vi "RandomInt64.vi"(10 "Min":i64, 11 "Max":i64) -> (3 "Random":i64)   [LabVIEW 2013]
doc: "Gives a random number between the two inputs, inclusive. \"Max\" can actually be smaller than \"Min,\" in this case, a random number [Max, Min] is given."
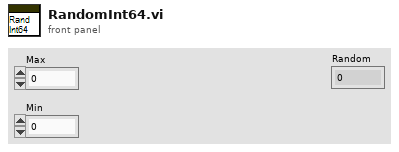
[diagram p1: front panel]
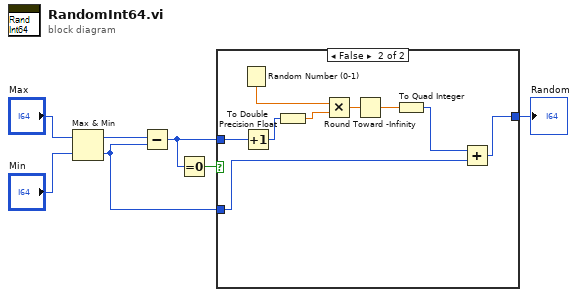
[diagram p0: block diagram]
diagram:
  n1 = Max & Min(x="Max", y="Min") -> (max(x,y)=w4:i64, min(x,y)=w1:i64)
  n2 = Subtract(x=w4, y=w1) -> (x-y=w3:i64)
  n3 = Equal To 0?(x=w3) -> (x = 0?=w2:bool)
  n4 = case shown="False" w2 {
    tunnel: [w8 w16] -> w7
    tunnel: w3 -> [_ w10]
    tunnel: w1 -> [w8 w9]
    frame True {
    }
    frame False {
      n5 = Random Number (0-1)() -> (number: 0 to 1=w17:dbl)
      n6 = Increment(x=w10) -> (x+1=w15:i64)
      n7 = To Double Precision Float(number=w15) -> (double precision float=w14:dbl)
      n8 = Multiply(x=w17, y=w14) -> (x*y=w13:dbl)
      n9 = Round Toward -Infinity(1:w13) -> (0:w12:dbl)
      n10 = To Quad Integer(1:w12) -> (0:w11:i64)
      n11 = Add(x=w11, y=w9) -> (x+y=w16:i64)
    }
  }
  "Random" <- w7
